vi "đèn giao thông.vi"() -> ()   [LabVIEW 2020]
panel:
  in  "stop":bool
  out "do 2":bool
  out "vang 2":bool
  out "xanh 2":bool
  out "do":bool
  out "vang":bool
  out "xanh":bool
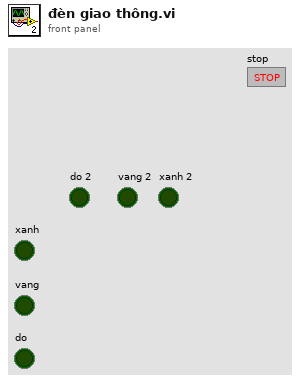
[diagram p1: front panel]
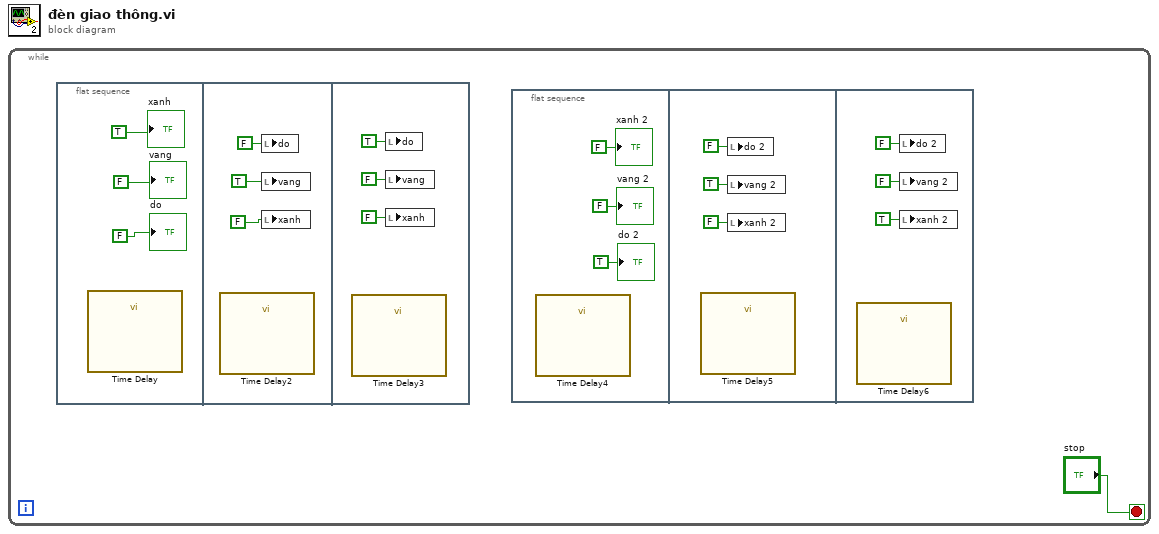
[diagram p0: block diagram]
diagram:
  n1 = while {
    stop <- "stop" stop-if-true
    n2 = flat-sequence {
      frame #0 {
        n3 = call "Time Delay"() -> ()  [unwired: 11 in, 1 out]
        "xanh" <- TRUE ("do")
        "vang" <- FALSE ("do")
        "do" <- FALSE ("do")
      }
      frame #1 {
        n4 = call "Time Delay2"() -> ()  [unwired: 11 in, 1 out]
        n5 = local write "do"(FALSE ("do")) -> ()
        n6 = local write "vang"(TRUE ("do")) -> ()
        n7 = local write "xanh"(FALSE ("do")) -> ()
      }
      frame #2 {
        n8 = call "Time Delay3"() -> ()  [unwired: 11 in, 1 out]
        n9 = local write "do"(TRUE ("do")) -> ()
        n10 = local write "vang"(FALSE ("vang")) -> ()
        n11 = local write "xanh"(FALSE ("xanh")) -> ()
      }
    }
    n12 = flat-sequence {
      frame #0 {
        n13 = call "Time Delay4"() -> ()  [unwired: 11 in, 1 out]
        "xanh 2" <- FALSE ("xanh 2")
        "vang 2" <- FALSE ("vang 2")
        "do 2" <- TRUE ("do 2")
      }
      frame #1 {
        n14 = call "Time Delay5"() -> ()  [unwired: 11 in, 1 out]
        n15 = local write "do 2"(FALSE ("do 2")) -> ()
        n16 = local write "vang 2"(TRUE ("vang 2")) -> ()
        n17 = local write "xanh 2"(FALSE ("xanh 2")) -> ()
      }
      frame #2 {
        n18 = call "Time Delay6"() -> ()  [unwired: 11 in, 1 out]
        n19 = local write "do 2"(FALSE ("do 2")) -> ()
        n20 = local write "vang 2"(FALSE ("vang 2")) -> ()
        n21 = local write "xanh 2"(TRUE ("xanh 2")) -> ()
      }
    }
  }
